vi "Stop Sequence.vi"(8 "error in (no error)":errorcluster, 10 "Sequence Name":string, 11 "Session Ref in":T1) -> (0 "error out":errorcluster, 2 "Sequence Name out":string, 3 "Session Ref out":T1)   [LabVIEW 2020, in "NI_VS Sequence Execution Interface.lvlib"]
doc: "Stops a real-time sequence in an NI VeriStand stimulus profile session, which causes the sequence to skip to the clean-up section. If you want to skip clean-up tasks, use the Abort Sequence VI."
uses:
  <vilib>/NI VeriStand/Execution/SequenceExecutionInterface/NI_VS Sequence Execution Interface.lvlib
  <vilib>/NI VeriStand/Execution/SequenceExecutionInterface/Stimulus Profile Session Ref.ctl
  NationalInstruments.VeriStand.ClientAPI
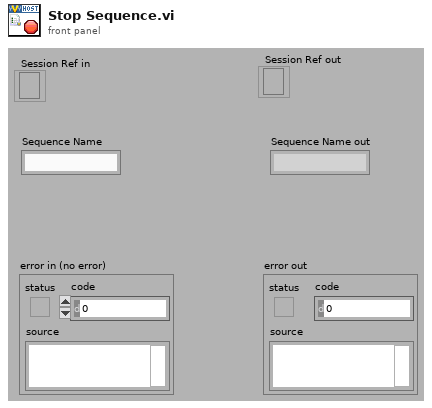
[diagram p1: front panel]
types:
  T1 = typedef "NI_VS Sequence Execution Interface.lvlib/Stimulus Profile Session Ref.ctl" = refnum<k24>
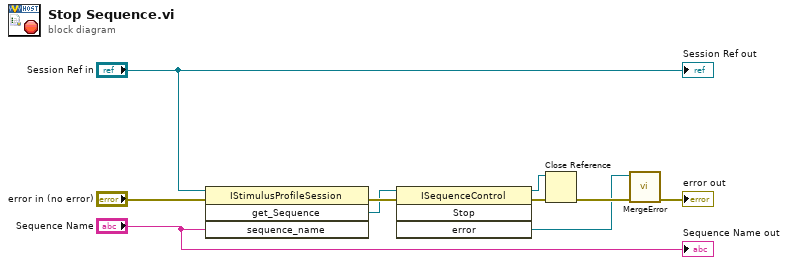
[diagram p0: block diagram]
diagram:
  n1 = invoke class="IStimulusProfileSession" method="get_Sequence"(reference="Session Ref in", error in="error in (no error)", "sequence_name"="Sequence Name") -> (error out=w10:errorcluster, "get_Sequence"=w7:refnum<k24>)  [unwired: 1 in, 2 out]
  n2 = invoke class="ISequenceControl" method="Stop"(reference=w7, error in=w10) -> (reference out=w5:refnum<k24>, error out=w6:errorcluster, "error"=w1:refnum<k24>)  [unwired: 2 in, 1 out]
  n3 = Close Reference(reference=w5, error in (no error)=w6) -> (error out=w3:errorcluster)
  n4 = call <vilib>:"MergeError.vi"("error in (no error)"=w3, "Error"=w1) -> ("error out"=→"error out":errorcluster)  [unwired: 9 out]
  "Session Ref out" <- "Session Ref in"
  "Sequence Name out" <- "Sequence Name"
